vi "DBL[1D]小数与整数（圆整）.vi"(11 "输入":dbl[](array[numeric])) -> (2 "小数部分":dbl[](array[numeric]), 3 "整数部分":dbl[](array[numeric]))   [LabVIEW 2012]
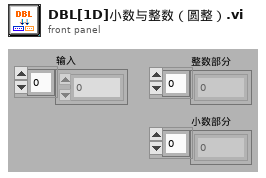
[diagram p1: front panel]
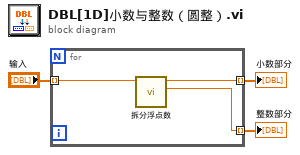
[diagram p0: block diagram]
diagram:
  n1 = for {
    tunnel: "输入" -> [w6] mode=indexing
    tunnel: [w5] -> w2 mode=indexing
    tunnel: [w4] -> w1 mode=indexing
    n2 = call-poly "拆分浮点数.vi"("输入"=w6) -> ("小数部分"=w4:dbl, "整数部分"=w5:dbl)  [unwired: 9 in]
  }
  "整数部分" <- w1
  "小数部分" <- w2
